vi "Pre Launch Init.vi"(11 "UI Main Startup in":refnum<class "UI Main Startup.lvclass">) -> (0 "error out":errorcluster, 3 "UI Main Startup out":refnum<class "UI Main Startup.lvclass">)   [LabVIEW 2020, in "UI Main Startup.lvlib" / "UI Main Startup.lvclass"]
doc: "(<B>Filename</B>: Actor Framework.lvlib:Actor.lvclass:Pre Launch Init.vi)\n\nDefines behavior that occurs after the Launch Nested Actor method is invoked but before the actor's Actor Core method begins running.\n\nBy default, this method does nothing. A descendant class may override it to define behavior."
uses:
  UI Main Startup.lvclass
  UI Main Startup.lvclass/UI Main Startup.ctl
  <vilib>/ActorFramework/Actor/Actor.lvclass
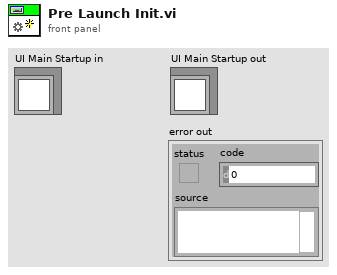
[diagram p1: front panel]
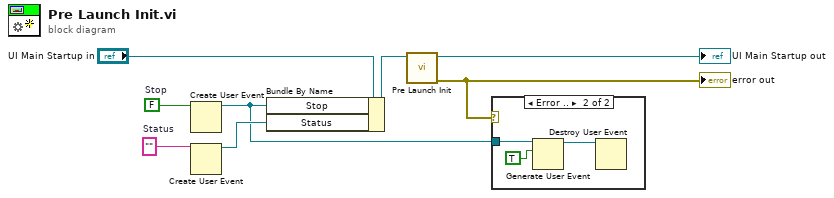
[diagram p0: block diagram]
diagram:
  w6 = ""  # Status
  w7 = FALSE  # Stop
  n1 = Create User Event(user event datatype=w7) -> (user event=w1:refnum<user-event>)  [unwired: 1 in, 1 out]
  n2 = Create User Event(user event datatype=w6) -> (user event=w3:refnum<user-event>)  [unwired: 1 in, 1 out]
  n3 = Bundle By Name(cluster="UI Main Startup in", "Stop"=w1, "Status"=w3) -> (w4:refnum<class "UI Main Startup.lvclass">)
  n4 = call-parent "Pre Launch Init.vi"("Actor in"=w4) -> ("error out"=w2:errorcluster, "Actor out"=→"UI Main Startup out":refnum<class "UI Main Startup.lvclass">)  [unwired: 9 in]
  "error out" <- w2
  n5 = case shown="Error .." w2 {
    tunnel: w1 -> [_ w11]
    frame No Error {
    }
    frame Error {
      n6 = Generate User Event(user event=w11, event data cluster=TRUE ("event data")) -> (user event out=w10:refnum<user-event>)  [unwired: 2 in, 1 out]
      n7 = Destroy User Event(user event=w10) -> ()  [unwired: 1 in, 1 out]
    }
  }
